vi "Send Tags.vi"(8 "error in (no error)":errorcluster, 11 "Logger in.lvclass":refnum<class "Logger.lvclass">) -> (0 "error out":errorcluster, 3 "Logger out.lvclass":refnum<class "Logger.lvclass">)   [LabVIEW 2017, in "Logger.lvclass"]
uses:
  Logger.lvclass
  Logger.lvclass/Logger.ctl
  <vilib>/TagLibrary/TagCluster.ctl
  <vilib>/TagLibrary/DataType.ctl
  <vilib>/TagLibrary/TagLibrary.lvlib
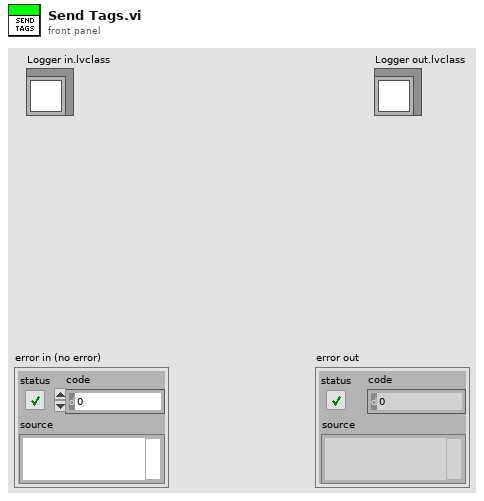
[diagram p1: front panel]
types:
  T1 = typedef "TagLibrary.lvlib/TagCluster.ctl" = cluster{"tag reference":refnum<k21>, "value":variant, "timestamp":timestamp, "data type":T2}
  T2 = typedef "TagLibrary.lvlib/DataType.ctl" = enum32{"Double", "Integer", "String"}
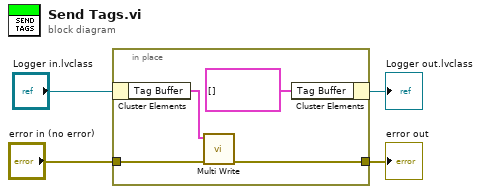
[diagram p0: block diagram]
diagram:
  n1 = in-place {
    in-place-border: "error in (no error)" -> [w6]
    in-place-border: [w5] -> w1
    n2 = in-place-cluster #1("Logger in.lvclass") -> ("Tag Buffer"=w7:T1[])
    n3 = call <vilib>:"Multi Write.vi"("tag clusters"=w7, "error in (no error)"=w6) -> ("error out"=w5:errorcluster)  [unwired: 7 in, 1 out]
    n4 = in-place-cluster #1("Tag Buffer"=T1[] []) -> (→"Logger out.lvclass":refnum<class "Logger.lvclass">)
  }
  "error out" <- w1
